vi "sv_Convert Even Angle Signal to Waveform.vi"(0 "even-angle signals":cluster{"r0":dbl, "dr":dbl, "Y":dbl[]}[](array[cluster]), 1 "even-angle channel info":T1[](array[typedef]) {"channel info"."pregain" format="%.2f"; "channel info"."weighting filter" items=["Linear", "A-weighting", "B-weighting", "C-weighting", "ITU-R 468-4", "Dolby", "CCITT", "C-message", "Wb", "Wc", "Wd", "We", "Wf", "Wh", "Wj", "Wk", "Wm", "AES17 20 kHz lowpass", "AES17 40 kHz lowpass", "AES17 20 kHz highpass", "AES17 40 kHz highpass"]; "channel info"."dB reference" format="%^.1e"; "channel info"."engineering units" items=["custom..."=0, "V"=1, "A"=21, "C"=30, "pC"=31, "s"=32, "-"=29, "Pa"=2, "N"=20, "g"=3, "m/s^2"=4, "m/s"=5, "m"=6, "mm/s"=12, "mm"=13, "micron/s"=14, "micron"=15, "in/s^2"=7, "in/s"=8, "in"=9, "mil/s"=10, "mil"=11, "rad/s^2"=16, "rad/s"=17, "rad"=18, "deg/s^2"=26, "deg/s"=27, "deg"=28, "RPM"=22, "cycle/s^2"=23, "Hz"=24, "cycle"=25, "strain"=19]; "channel info"."sensor sensitivity" format="%#_5f"}, 2 "reset? (F)":bool, 3 "stopband attenuation [dB]":dbl=96.0, 5 "new sample phase":dbl[](array[numeric]) format="%.2f", 7 "new dt":dbl, 9 "new t0":timestamp, 11 "error in (no error)":errorcluster) -> (4 "Waveform":waveform(dbl)[](array[waveform]), 15 "error out":errorcluster)   [LabVIEW 2017, in "SoundVib_ContSweptSine.lvlib"]
doc: "Converts an even-time-spaced scaled signal to an even-angle-spaced signal by resampling the acquired signal. The output signal is synchronous to the rotational speed with a constant number of samples per revolution. The data type you wire to the <B>scaled signal [EU]</B> input determines the polymorphic instance to use."
uses:
  <vilib>/addons/Sound and Vibration/svt_Continuous Swept Sine/SoundVib_ContSweptSine.lvlib
  <vilib>/addons/_NISVFA/_Shared subVIs/Controls/svc_Resampled Channel Info.ctl
  <vilib>/addons/_NISVFA/_Shared subVIs/Controls/svc_Channel Info.ctl
  <vilib>/addons/_NISVFA/_Shared subVIs/Controls/svc_Engineering Units Text Ring.ctl
  <vilib>/addons/_NISVFA/_Shared subVIs/Controls/svc_Weighting Filter Text Ring.ctl
  <vilib>/addons/_NISVFA/_Shared subVIs/Common/svc_Set SV Channel Info (variant).vi
  <vilib>/addons/_NISVFA/_Shared subVIs/Common/SVL Set dB Reference (variant).vi
  <vilib>/addons/_NISVFA/_Shared subVIs/Common/svc_Engineering Units to Unit Label.vi
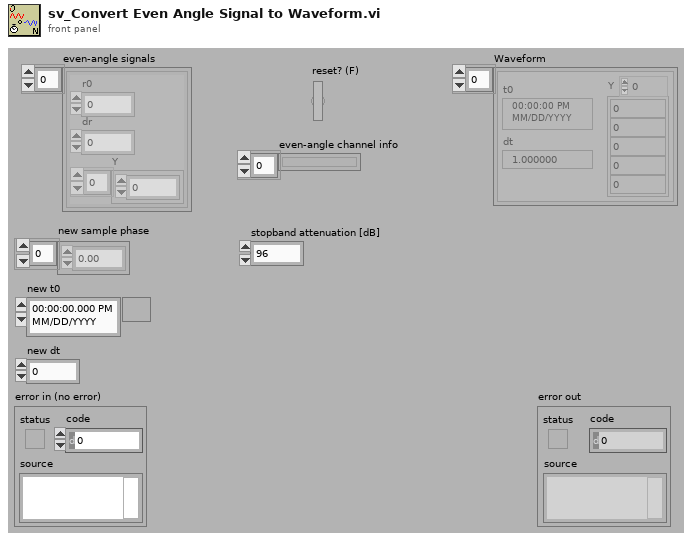
[diagram p1: front panel]
types:
  T1 = typedef "svc_Resampled Channel Info.ctl" = cluster{"channel name":string, "description":string, " channel info":T2}
  T2 = typedef "svc_Channel Info.ctl" = cluster{"sensor sensitivity":dbl, "engineering units":T3, "dB reference":dbl, "custom label":string, "weighting filter":T4, "pregain":dbl}
  T3 = typedef "svc_Engineering Units Text Ring.ctl" = u16
  T4 = typedef "svc_Weighting Filter Text Ring.ctl" = u16
  T5 = typedef "OAT Resample Filter Prototype.ctl" = cluster{"left wing":dbl[], "increment":dbl[], "max dec":i32, "timing jitter":enum32{"Interpolation", "Rounding"}, "band limiting?":bool}
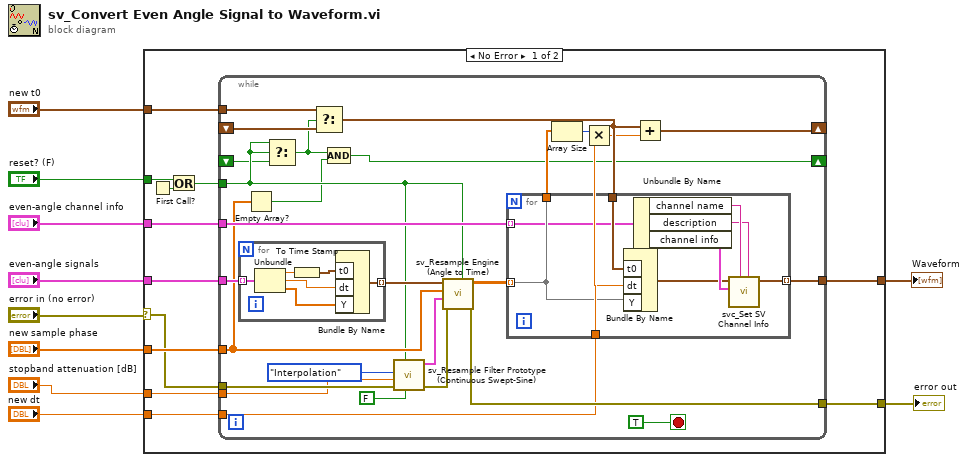
[diagram p0: block diagram]
diagram:
  n1 = case shown="No Error" "error in (no error)" {
    selector: "error in (no error)" -> [w18 w65]
    tunnel: [w22 w65] -> w10
    tunnel: "reset? (F)" -> [w20 _]
    tunnel: "new dt" -> [w17 _]
    tunnel: "new sample phase" -> [w19 _]
    tunnel: "new t0" -> [w15 _]
    tunnel: [w13 _] -> w1
    tunnel: "stopband attenuation [dB]" -> [w14 _]
    tunnel: "even-angle signals" -> [w12 _]
    tunnel: "even-angle channel info" -> [w11 _]
    frame No Error {
      n2 = First Call?() -> (First Call?: T/F=w21:bool)
      n3 = Or(x=w20, y=w21) -> (x .or. y?=w16:bool)
      n4 = while {
        tunnel: [w48] -> w22
        tunnel: w19 -> [w28]
        tunnel: w18 -> [w44]
        tunnel: w17 -> [w43]
        tunnel: w16 -> [w27]
        tunnel: w15 -> [w42]
        tunnel: [w38] -> w13
        tunnel: w14 -> [w36]
        shift-right: [w34] -> _
        shift-left: _ -> [w33]
        tunnel: w12 -> [w31]
        tunnel: w11 -> [w29]
        shift-right: [w23] -> _
        shift-left: _ -> [w26]
        stop <- TRUE stop-if-true
        n5 = for {
          tunnel: w31 -> [w55] mode=indexing
          tunnel: [w50] -> w30 mode=indexing
          n6 = Unbundle(w55) -> ("r0"=w54:dbl, "dr"=w52:dbl, "Y"=w51:dbl[])
          n7 = To Time Stamp(1:w54) -> (0:w53:timestamp)
          n8 = Bundle By Name("t0"=w53, "dt"=w52, "Y"=w51) -> (w50:waveform(dbl))  [unwired: 1 in]
        }
        n9 = Empty Array?(array=w28) -> (empty?=w24:bool)
        n10 = Select(t=w27, s=w27, f=w26) -> (s? t:f=w25:bool)
        n11 = Select(t=w42, s=w25, f=w33) -> (s? t:f=w41:timestamp)
        n12 = Compound Arithmetic op=AND(w25, w24) -> (w23:bool)
        n13 = call <vilib>:"sv_Resample Filter Prototype (Continuous Swept-Sine).vi"("alias free"=FALSE ("alias protect in final transition"), "reset? (True)"=w27, "error in (no error)"=w44, "stop band attenuation [dB]"=w36, "timing jitter"=enum32{"Interpolation", "Rounding"}."Interpolation") -> ("error out"=w45:errorcluster, "filter prototype"=w47:T5)  [unwired: 4 in, 1 out]
        n14 = call <vilib>:"sv_Resample Engine (Angle to Time).vi"("reset? (True)"=w27, "error in (no error)"=w45, "filter prototype"=w47, "time"=w28, "scaled signals (EU)"=w30) -> ("error out"=w48:errorcluster, "Y"=w32:dbl[][])  [unwired: 5 out]
        n15 = for {
          tunnel: w43 -> [w64]
          tunnel: w41 -> [w63]
          tunnel: [w62] -> w39
          tunnel: [w57] -> w38 mode=indexing
          tunnel: w32 -> [w62] mode=indexing
          tunnel: w29 -> [w56] mode=indexing
          n16 = Bundle By Name("t0"=w63, "dt"=w64, "Y"=w62) -> (w58:waveform(dbl))  [unwired: 1 out]
          n17 = Unbundle By Name(w56) -> ("channel name"=w61:string, "description"=w60:string, "channel info"=w59:T2)
          n18 = call <vilib>:"svc_Set SV Channel Info.vi"("channel description"=w60, "channel name"=w61, "channel info"=w59, "scaled signal in"=w58) -> ("scaled signal out"=w57:waveform(dbl))  [unwired: 1 in, 6 out]
        }
        n19 = Array Size(array=w39) -> (size(s)=w40:i32)
        n20 = Multiply(x=w40, y=w43) -> (x*y=w37:dbl)
        n21 = Add(x=w41, y=w37) -> (x+y=w34:timestamp)
      }
    }
    frame Error {
    }
  }
  "error out" <- w10
  "Waveform" <- w1
